vi "Backup Plot Name.vi"(8 "error in (no error)":errorcluster, 11 "3D Contour.lvclass in":refnum<class "3D Contour.lvclass">) -> (0 "error out":errorcluster, 3 "3D Contour.lvclass out":refnum<class "3D Contour.lvclass">)   [LabVIEW 2017, in "3D Contour.lvclass"]
uses:
  <vilib>/Math Plots/3D Math Plots/3D Contour/3D Contour/3D Contour.lvclass
  e:/builds/penguin/labview/branches/2017/dev/dist/vi.lib/Math Plots/3D Math Plots/3D Plot/3D Plot/3D Plot.lvclass
  <vilib>/Math Plots/3D Math Plots/3D Contour/3D Contour/3D Contour.lvclass/3D Contour.ctl
  <vilib>/Math Plots/3D Math Plots/3D Plot/3D Plot/3D Plot.lvclass
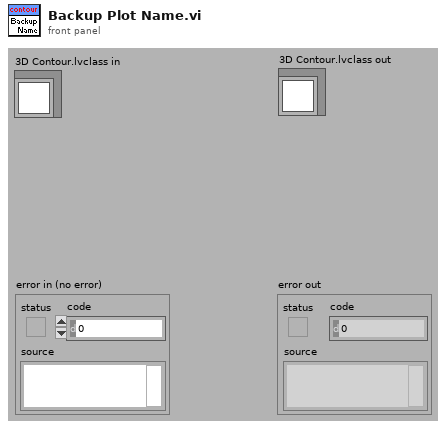
[diagram p1: front panel]
types:
  T1 = typedef "3D Plot.lvclass/Property Cluster.ctl" = cluster{"Graph Property":T2, "Light Property":T6, "Axis Property":T8, "Value Pair Property":T15, "Format Property":T17, "Cursor Property Array":T18, "Appearance Property":T27}
  T2 = typedef "3D Plot.lvclass/Graph Property.ctl" = cluster{"General Property":T3, "View Property":T4, "Grid Plane":T5}
  T3 = typedef "3D Plot.lvclass/General Property.ctl" = cluster{"Plot Area Color":u32, "Fast Draw?":bool, "Clip Data?":bool}
  T4 = typedef "3D Plot.lvclass/View Property.ctl" = cluster{"Projection Mode":enum16{"Orthographic", "Perspective"}, "View Direction":enum32{"Towards X-Y Plane", "Towards X-Z Plane", "Towards Y-Z Plane", "User Defined"}, "User Defined View Direction":cluster{"View Latitude":sgl, "View Longitude":sgl, "View Distance":sgl}}
  T5 = typedef "3D Plot.lvclass/Grid Plane.ctl" = cluster{"Grid Plane Visible":cluster{"Draw Grid Plane X-Y":bool, "Draw Grid Plane Y-Z":bool, "Draw Grid Plane X-Z":bool}, "Grid Antialiasing":bool, "Grid Frame Color":u32}
  T6 = typedef "3D Plot.lvclass/Light Property.ctl" = cluster{"Enable Lighting?":bool, "Ambient Color":u32, "Light Array":T7[]}
  T7 = typedef "3D Plot.lvclass/Light Specific.ctl" = cluster{"Enable Light?":bool, "Light Color":u32, "Light Latitude":sgl, "Light Longitude":sgl, "Light Distance":sgl, "Attenuation":enum16{"None", "Linear", "Quadratic"}}
  T8 = typedef "3D Plot.lvclass/Axis Property.ctl" = cluster{"Caption Property":T9, "Label Property":T10, "Range Property":T11, "Grid Property":T13, "Ticks Property":T14}
  T9 = typedef "3D Plot.lvclass/Caption Property.ctl" = cluster{"Show Caption":cluster{"Show Normal X Caption":bool, "Show Normal Y Caption":bool, "Show Normal Z Caption":bool, "Show Opposite X Caption":bool, "Show Opposite Y Caption":bool, "Show Opposite Z Caption":bool}, "Caption Color":cluster{"Caption Color X":u32, "Caption Color Y":u32, "Caption Color Z":u32}, "Caption Size":cluster{"Caption Size X":u16, "Caption Size Y":u16, "Caption Size Z":u16}, "Caption String":cluster{"Caption X":string, "Caption Y":string, "Caption Z ":string}}
  T10 = typedef "3D Plot.lvclass/Label Property.ctl" = cluster{"Show Label":cluster{"Show Normal X Label":bool, "Show Normal Y Label":bool, "Show Normal Z Label":bool, "Show Opposite X Label":bool, "Show Opposite Y Label":bool, "Show Opposite Z Label":bool}, "Label Color":cluster{"Label Color X":u32, "Label Color Y":u32, "Label Color Z":u32}, "Label Size":cluster{"Label Size X":u16, "Label Size Y":u16, "Labe Size Z":u16}}
  T11 = typedef "3D Plot.lvclass/Range Property.ctl" = cluster{"Range Cluster":T12, "Auto Range":cluster{"Auto Range X":bool, "Auto Range Y":bool, "Auto Range Z":bool}, "Inverted":cluster{"Inverted X":bool, "Inverted Y":bool, "Inverted Z":bool}, "Logarithm":cluster{"Logarithm X":bool, "Logarithm Y":bool, "Logarithm Z":bool}}
  T12 = typedef "3D Plot.lvclass/Range Clusters.ctl" = cluster{"X Range":cluster{"Max X":sgl, "Min X":sgl}, "Y Range":cluster{"Max Y":sgl, "Min Y":sgl}, "Z Range":cluster{"Max Z":sgl, "Min Z":sgl}}
  T13 = typedef "3D Plot.lvclass/Grid Property.ctl" = cluster{"Major Grid Visible":cluster{"Draw Major Grid X":bool, "Draw Major Grid Y":bool, "Draw Major Grid Z":bool}, "Major Grid Color":cluster{"Major Grid Color X":u32, "Major Grid Color Y":u32, "Major Grid Color Z":u32}, "Minor Grid Visible":cluster{"Draw Minor Grid X":bool, "Draw Minor Grid Y":bool, "Draw Minor Grid Z":bool}, "Minor Grid Color":cluster{"Minor Grid Color X":u32, "Minor Grid Color Y":u32, "Minor Grid Color Z":u32}}
  T14 = typedef "3D Plot.lvclass/Tick Property.ctl" = cluster{"Major Tick Visible":cluster{"Draw Major Tick X":bool, "Draw Major Tick Y":bool, "Draw Major Tick Z":bool}, "Major Tick Color":cluster{"Major Tick Color X":u32, "Major Tick Color Y":u32, "Major Tick Color Z":u32}, "Major Count":cluster{"Major Count X":u16, "Major Count Y":u16, "Major Count Z":u16}, "Minor Tick Visible":cluster{"Draw Minor Tick X":bool, "Draw Minor Tick Y":bool, "Draw Minor Tick Z":bool}, "Minor Tick Color":cluster{"Minor Tick Color X":u32, "Minor Tick Color Y":u32, "Minor Tick Color Z":u32}, "Minor Count":cluster{"Minor Count X":u16, "Minor Count Y":u16, "Minor Count Z":u16}}
  T15 = typedef "3D Plot.lvclass/Value Pair Property.ctl" = T16[]
  T16 = typedef "3D Plot.lvclass/Value Pair Cluster.ctl" = cluster{"Value Pair Array":cluster{"Value":sgl, "Name":string}[], "Show Tick":bool, "Show Grid":bool, " Label Mode":enum16{"Name", "Value", "None"}}
  T17 = typedef "3D Plot.lvclass/Format Property.ctl" = string[]
  T18 = typedef "3D Plot.lvclass/Cursor Property Array.ctl" = T19[]
  T19 = typedef "3D Plot.lvclass/Cursor Property.ctl" = cluster{"Cursor Visible":bool, "Cursor Enable":bool, "Cursor Position":T20, "Cursor Point":T21, "Cursor Line":T23, "Cursor Plane":T25, "Cursor Text":T26}
  T20 = typedef "3D Plot.lvclass/Cursor Position.ctl" = cluster{"Cursor Plot ID":i32, "Cursor X":sgl, "Cursor Y":sgl, "Cursor Z":sgl, "Cursor Snap To":enum16{"Fixed", "Nearest Plot", "Snap to Plot"}}
  T21 = typedef "3D Plot.lvclass/Cursor Point.ctl" = cluster{"Cursor Point Color":u32, "Cursor Point Size":sgl, "Cursor Point Style":T22}
  T22 = typedef "3D Plot.lvclass/Sprite Type.ctl" = enum16{"None", "Empty Square", "Solid Square", "Empty Diamond", "Solid Diamond", "Empty Circle", "Solid Circle", "Asterisk", "Bold X", "Wireframe Sphere", "Solid Sphere", "Wireframe Cube", "Solid Cube"}
  T23 = typedef "3D Plot.lvclass/Cursor Line.ctl" = cluster{"Cursor Line Color":u32, "Cursor Line Width":sgl, "Cursor Line Style":T24}
  T24 = typedef "3D Plot.lvclass/Line Type.ctl" = enum16{"None", "Solid", "Dash", "Dot", "Dash Dot"}
  T25 = typedef "3D Plot.lvclass/Cursor Plane.ctl" = cluster{"Cursor Plane Color":u32, "Cursor Plane Opacity":sgl, "Draw Cursor Plane X-Z":bool, "Draw Cursor Plane Y-Z":bool, "Draw Cursor Plane X-Y":bool}
  T26 = typedef "3D Plot.lvclass/Cursor Text.ctl" = cluster{"Cursor Text":string, "Cursor Text Size":u16, "Cursor Show Position":bool, "Cursor Show Name":bool, "Cursor Text Color":u32, "Background Color":u32, "Background Opacity":sgl}
  T27 = typedef "3D Plot.lvclass/Apearance Property.ctl" = cluster{"Visibility":T28, "Active Index":cluster{"Active Plot":i32, "Active Cursor":i32, "Active Axis":enum16{"X-axis", "Y-axis", "Z-axis"}, "Active Value Pair":enum16{"X-axis", "Y-axis", "Z-axis"}, "Active Light":enum16{"Light 0", "Light 1", "Light 2", "Light 3"}}, "Backup Data":cluster{"Plot Name":string[]}}
  T28 = typedef "3D Plot.lvclass/Item Visibility.ctl" = cluster{"Projection Palette":bool, "Color Ramp Palette":bool}
  T29 = typedef "3D Contour.lvclass/3D Contour Property Array.ctl" = T30[]
  T30 = typedef "3D Contour.lvclass/3D Contour Property.ctl" = cluster{"General Property":cluster{"Plot Name":string, "Coordinate System":enum16{"Cartesian", "Cylindrical", "Spherical"}, "Opacity":sgl}, "Projection Property":cluster{"Draw XY":bool, "Draw YZ":bool, "Draw XZ":bool}, "Plot Property":cluster{"Line Style":T24, "Line Width":sgl, "Line Color":u32, "Antialiasing":bool, "Color Ramp Cluster":T31}, "Contour Property":cluster{"Contour Type":enum16{"Contour", "Contour with surface"}, "Axis Basis":enum16{"X-Axis", "Y-Axis", "Z-Axis"}, "Level List":sgl[], "Level Mode":enum16{"Levels", "Interval", "Level List"}, "Levels":u16, "Interval":sgl}}
  T31 = typedef "3D Plot.lvclass/Color Ramp Cluster.ctl" = cluster{"Color Ramp Style":enum16{"None", "Shaded", "Color spectrum", "Grey scale", "Custom"}, "Color Ramp Array":u32[], "Color Ramp Index":i32[], "Interpolate?":bool, "Logarithm?":bool}
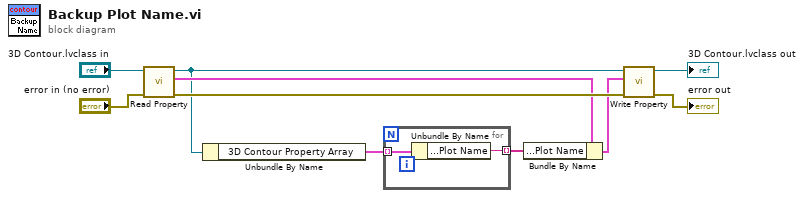
[diagram p0: block diagram]
diagram:
  n1 = call <vilib>:"Read Property.vi"("error in (no error)"="error in (no error)", "3D Plot.lvclass in"="3D Contour.lvclass in") -> ("error out"=w9:errorcluster, "Property Cluster"=w6:T1, "3D Plot.lvclass out"=w5:refnum<class "3D Contour.lvclass">)  [unwired: 7 out]
  n2 = Unbundle By Name(w5) -> ("3D Contour Property Array"=w10:T29)
  n3 = for {
    tunnel: w10 -> [w12] mode=indexing
    tunnel: [w11] -> w7 mode=indexing
    n4 = Unbundle By Name(w12) -> ("General Property.Plot Name"=w11:string)
  }
  n5 = Bundle By Name(cluster=w6, "Appearance Property.Backup Data.Plot Name"=w7) -> (w8:T1)
  n6 = call <vilib>:"Write Property.vi"("error in (no error)"=w9, "Property Cluster"=w8, "3D Plot.lvclass in"=w5) -> ("error out"=→"error out":errorcluster, "3D Plot.lvclass out"=→"3D Contour.lvclass out":refnum<class "3D Contour.lvclass">)  [unwired: 7 out]
